vi "Exemple_guider_3.vi"() -> ()   [LabVIEW 2018]
panel:
  in  "Choix":i8
  out "N-1":i8
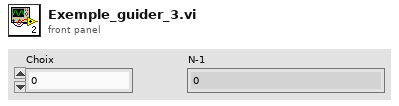
[diagram p1: front panel]
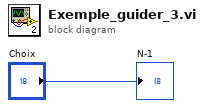
[diagram p0: block diagram]
diagram:
  "N-1" <- "Choix"
